vi "Facade.vi"(0 "Data In":T4, 2 "Display State In":T2, 3 "Container State":T3) -> (6 "Data Out":T4, 7 "Display State Out":T2, 8 "Action":T1)   [LabVIEW 2014, in "Electrode XCtl.xctl"]
uses:
  Electrode XCtl.xctl
  Data.ctl
  <vilib>/_xctls/Container State.ctl
  State.ctl
  <vilib>/_xctls/Action.ctl
  <vilib>/_xctls/XControlSupport.lvlib
panel:
  out "3":bool
  out "4":bool
  out "2":bool
  out "1":bool
  in  "Btn":bool
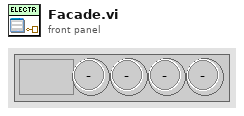
[diagram p1: front panel]
types:
  T1 = typedef "XControlSupport.lvlib/Action.ctl" = cluster{"Data Changed?":bool, "State Changed?":bool, "Action Name":string}
  T2 = typedef "Electrode XCtl.xctl/State.ctl" = cluster{"Numeric":dbl}
  T3 = typedef "XControlSupport.lvlib/Container State.ctl" = cluster{"Indicator?":bool, "Run Mode?":bool, " Refnum":refnum<vi>}
  T4 = typedef "Electrode XCtl.xctl/Data.ctl" = cluster{"Data":u16, "ElectrodeStates":cluster{"On_Off":bool, "Text":string}[], "ModOn":bool}
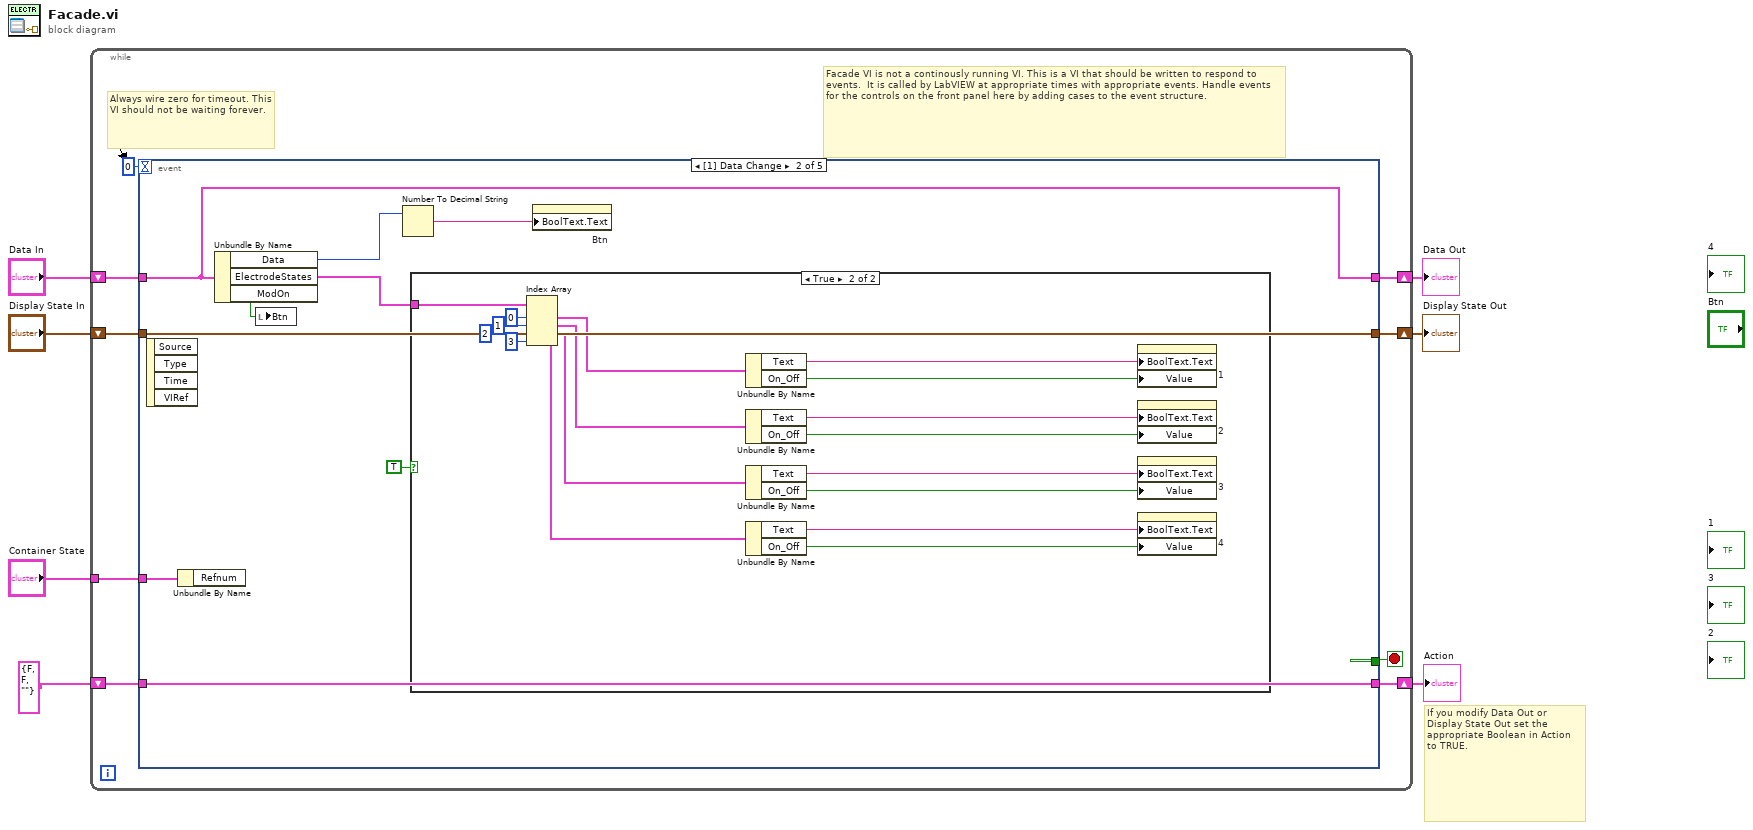
[diagram p0: block diagram]
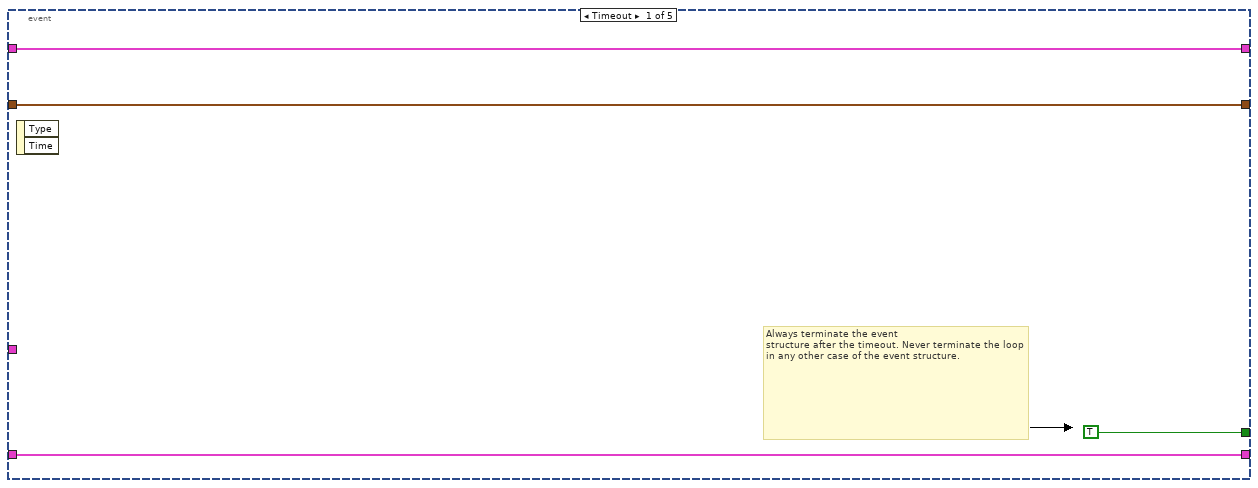
[diagram p2: hidden frame]
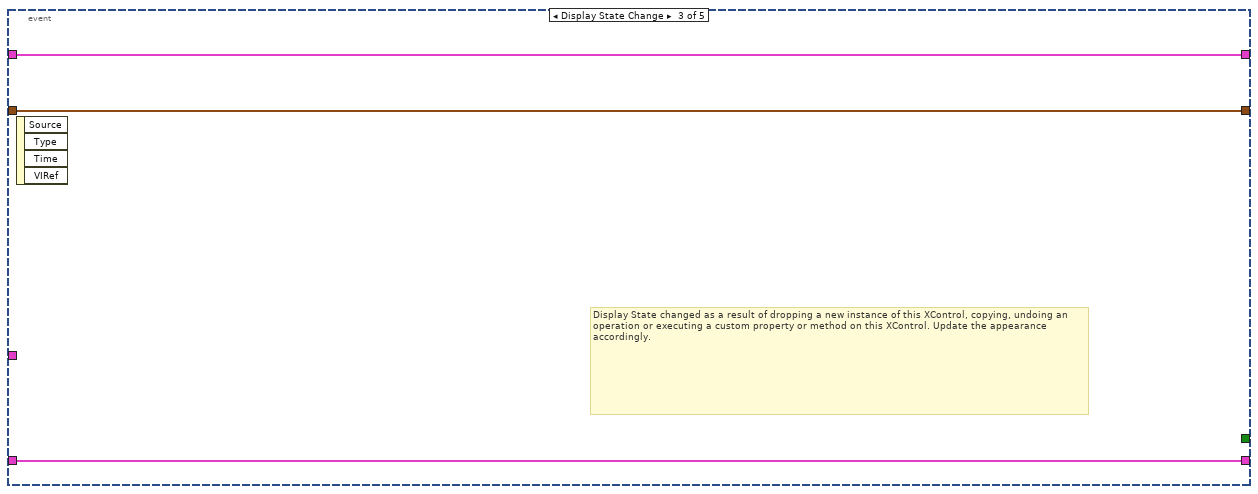
[diagram p4: hidden frame]
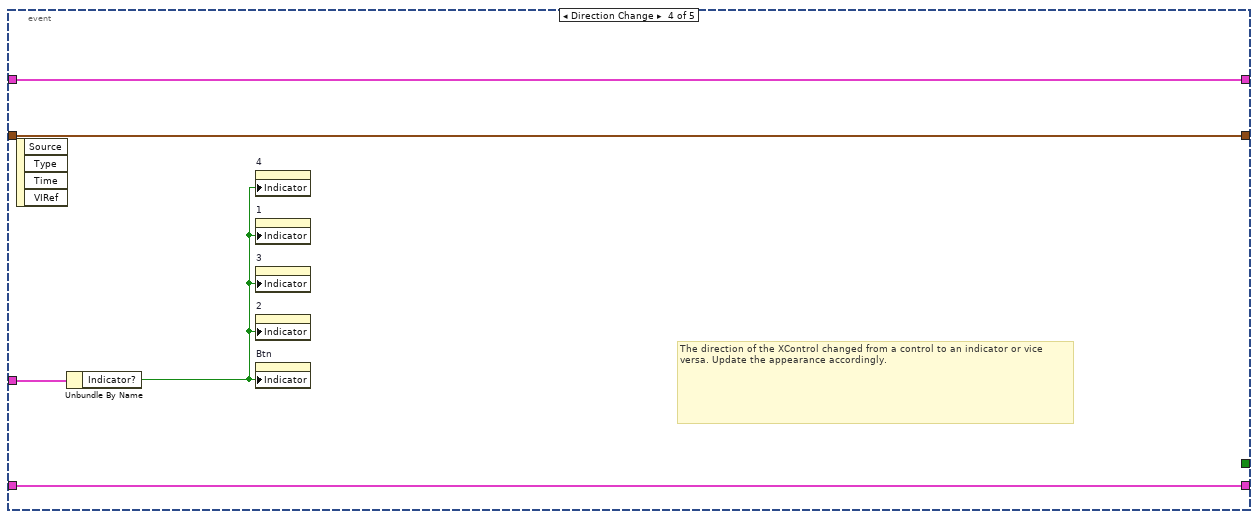
[diagram p5: hidden frame]
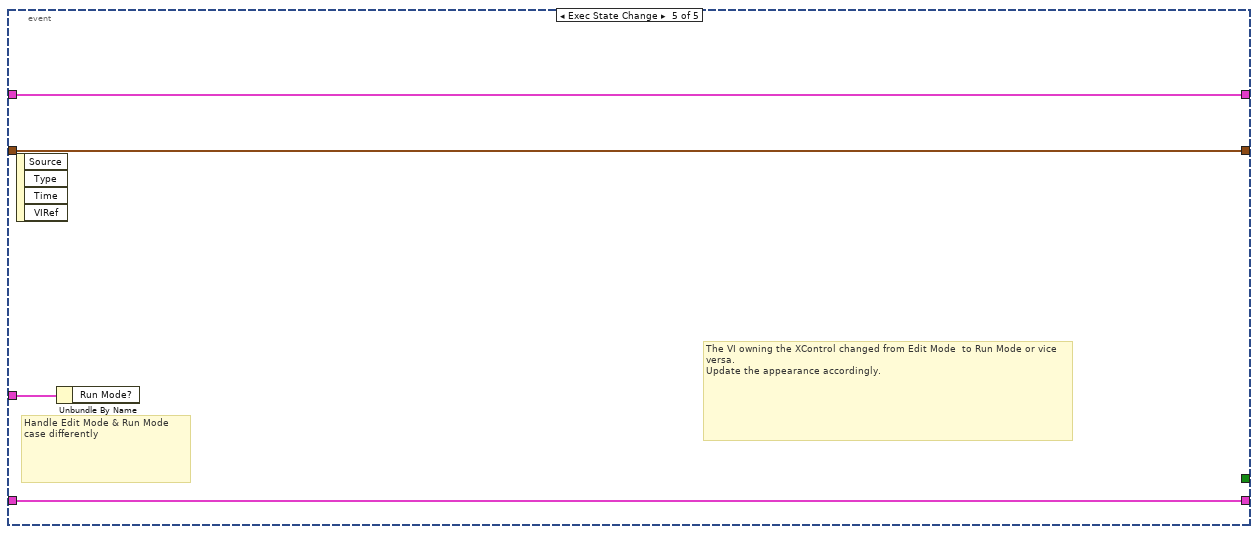
[diagram p6: hidden frame]
diagram:
  # "If you modify Data Out or\nDisplay State Out set the\nappropriate Boolean in Action\nto TRUE."
  n1 = while {
    shift-right: [w15] -> w4
    shift-left: "Display State In" -> [w16]
    tunnel: "Container State" -> [w12]
    shift-right: [w10] -> w7
    shift-left: "Data In" -> [w11]
    shift-right: [w8] -> w2
    shift-left: T1 {"Data Changed?"=FALSE, "State Changed?"=FALSE, "Action Name"=""} ("Action") -> [w9]
    stop <- w14 stop-if-true
    # "Facade VI is not a continously running VI. This is a VI that should be written to respond to events.  It is called by LabVIEW at appropriate times with appropriate events. Handle events for the controls on the front panel here by adding cases to the event structure."
    # "Always wire zero for timeout. This\nVI should not be waiting forever."
    n2 = event shown="[1] Data Change" {
      selector: _ -> [_ _ _ _ _]
      dyn-events: _ -> [_ _ _ _ _]
      timeout: 0 -> [_ _ _ _ _]
      tunnel: w16 -> [w18 w27 w49 w53 w57]
      tunnel: [w18 w27 w49 w53 w57] -> w15
      tunnel: [TRUE _ _ _ _] -> w14
      tunnel: w12 -> [_ w25 _ w54 w58]
      tunnel: w11 -> [w17 w28 w47 w52 w56]
      tunnel: [w17 w28 w47 w52 w56] -> w10
      tunnel: [w19 w29 w48 w51 w55] -> w8
      tunnel: w9 -> [w19 w29 w48 w51 w55]
      event Timeout {
        # "Always terminate the event\nstructure after the timeout. Never terminate the loop in any other case of the event structure."
        n3 = event-data() -> ()  [unwired: 1 in, 2 out]
      }
      event Data Change {
        n4 = event-data() -> ()  [unwired: 1 in, 4 out]
        n5 = Unbundle By Name(w25) -> ()  [unwired: 1 out]
        n6 = Unbundle By Name(w28) -> ("Data"=w26:u16, "ElectrodeStates"=w23:cluster{"On_Off":bool, "Text":string}[], "ModOn"=w24:bool)
        n7 = local write "Btn"(w24) -> ()
        n8 = Number To Decimal String(number=w26) -> (decimal integer string=w21:string)  [unwired: 1 in]
        n9 = case shown="True" TRUE {
          tunnel: w23 -> [_ w46]
          frame False {
          }
          frame True {
            n10 = Index Array(array=w46, index #1=0 ("index"), index #2=1 ("index"), index #3=2 ("index"), index #4=3 ("index")) -> (element #1=w41:cluster{"On_Off":bool, "Text":string}, element #2=w33:cluster{"On_Off":bool, "Text":string}, element #3=w32:cluster{"On_Off":bool, "Text":string}, element #4=w31:cluster{"On_Off":bool, "Text":string})
            n11 = Unbundle By Name(w41) -> ("Text"=w30:string, "On_Off"=w34:bool)
            n12 = Unbundle By Name(w33) -> ("Text"=w36:string, "On_Off"=w35:bool)
            n13 = Unbundle By Name(w32) -> ("Text"=w39:string, "On_Off"=w40:bool)
            n14 = Unbundle By Name(w31) -> ("Text"=w38:string, "On_Off"=w37:bool)
            n15 = property on="1" class="Bool (strict)"("BoolText.Text"=w30, "Value"=w34) -> ()  [unwired: 2 in, 2 out]
            n16 = property on="2" class="Bool (strict)"("BoolText.Text"=w36, "Value"=w35) -> ()  [unwired: 2 in, 2 out]
            n17 = property on="3" class="Bool (strict)"("BoolText.Text"=w39, "Value"=w40) -> ()  [unwired: 2 in, 2 out]
            n18 = property on="4" class="Bool (strict)"("BoolText.Text"=w38, "Value"=w37) -> ()  [unwired: 2 in, 2 out]
          }
        }
        n19 = property on="Btn" class="Bool (strict)"("BoolText.Text"=w21) -> ()  [unwired: 2 in, 2 out]
      }
      event Display State Change {
        # "Display State changed as a result of dropping a new instance of this XControl, copying, undoing an operation or executing a custom property or method on this XControl. Update the appearance accordingly."
        n20 = event-data() -> ()  [unwired: 1 in, 4 out]
      }
      event Direction Change {
        # "The direction of the XControl changed from a control to an indicator or vice versa. Update the appearance accordingly."
        n21 = event-data() -> ()  [unwired: 1 in, 4 out]
        n22 = Unbundle By Name(w54) -> ("Indicator?"=w50:bool)
        n23 = property on="4" class="Bool (strict)"("Indicator"=w50) -> ()  [unwired: 2 in, 2 out]
        n24 = property on="1" class="Bool (strict)"("Indicator"=w50) -> ()  [unwired: 2 in, 2 out]
        n25 = property on="3" class="Bool (strict)"("Indicator"=w50) -> ()  [unwired: 2 in, 2 out]
        n26 = property on="2" class="Bool (strict)"("Indicator"=w50) -> ()  [unwired: 2 in, 2 out]
        n27 = property on="Btn" class="Bool (strict)"("Indicator"=w50) -> ()  [unwired: 2 in, 2 out]
      }
      event Exec State Change {
        # "The VI owning the XControl changed from Edit Mode  to Run Mode or vice versa.\nUpdate the appearance accordingly."
        # "Handle Edit Mode & Run Mode\ncase differently"
        n28 = event-data() -> ()  [unwired: 1 in, 4 out]
        n29 = Unbundle By Name(w58) -> ()  [unwired: 1 out]
      }
    }
  }
  "Display State Out" <- w4
  "Data Out" <- w7
  "Action" <- w2
